vi "g_Joystick2.vi"(7 "Action":enum16{"initialize", "read", "write"}(ring), 9 "Buttons":bool[](array[boolean]), 10 "Axes":dbl[](array[numeric]), 11 "DebounceLength":i32=1) -> (1 "Buttons out":T2, 2 "Axes out":T1 {"Switch" format="%#_4g"; "Axis 2" format="%#_4g"; "Axis 1" format="%#_4g"; "Axis 0" format="%#_4g"}, 4 "Array":cluster{"DbArray":bool[]}[](array[cluster]))   [LabVIEW 2017]
uses:
  Ctrl Refs/JoyStick2.ctl
  Ctrl Refs/JoyStick2(Analog).ctl
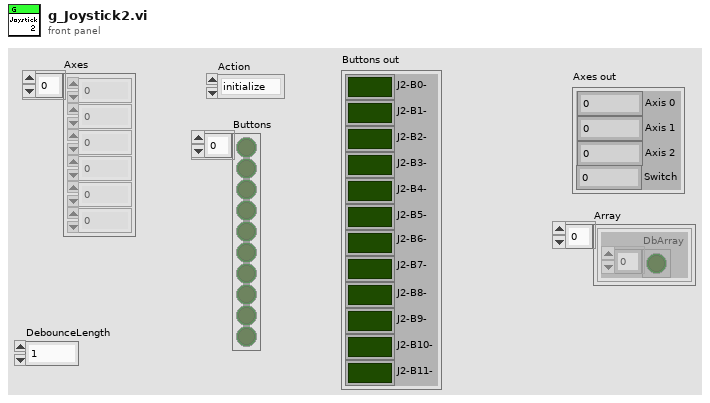
[diagram p1: front panel]
types:
  T1 = typedef "JoyStick2(Analog).ctl" = cluster{"Axis 0":dbl, "Axis 1":dbl, "Axis 2":dbl, "Switch":dbl}
  T2 = typedef "JoyStick2.ctl" = cluster{"J2-B0-":bool, "J2-B1-":bool, "J2-B2-":bool, "J2-B3-":bool, "J2-B4-":bool, "J2-B5-":bool, "J2-B6-":bool, "J2-B7-":bool, "J2-B8-":bool, "J2-B9-":bool, "J2-B10-\n":bool, "J2-B11-":bool}
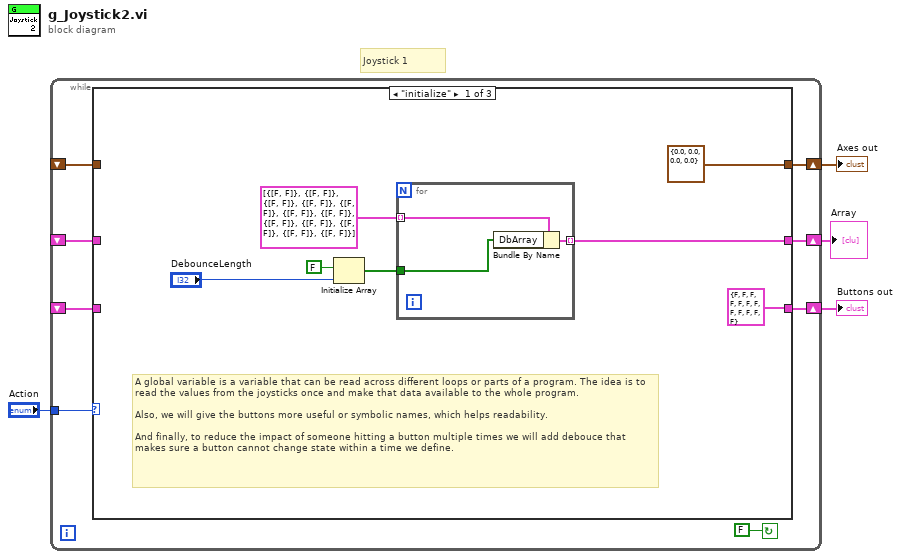
[diagram p0: block diagram]
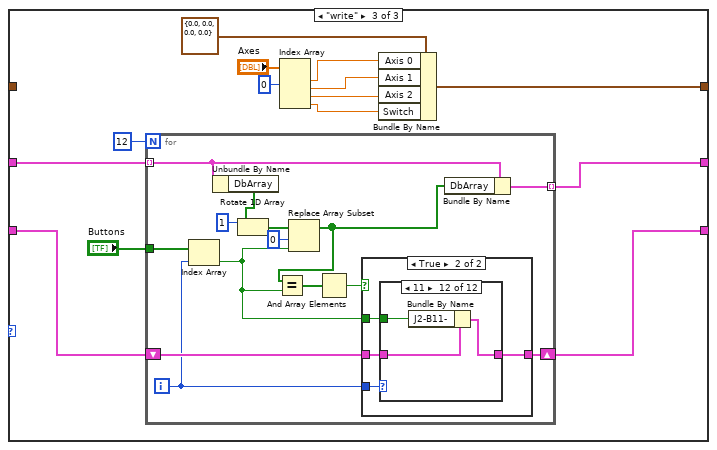
[diagram p3: hidden frame]
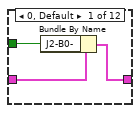
[diagram p5: hidden frame]
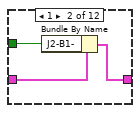
[diagram p6: hidden frame]
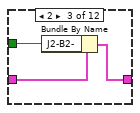
[diagram p7: hidden frame]
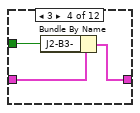
[diagram p8: hidden frame]
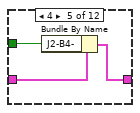
[diagram p9: hidden frame]
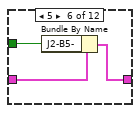
[diagram p10: hidden frame]
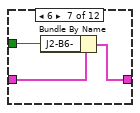
[diagram p11: hidden frame]
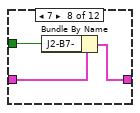
[diagram p12: hidden frame]
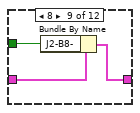
[diagram p13: hidden frame]
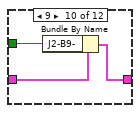
[diagram p14: hidden frame]
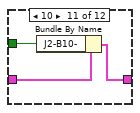
[diagram p15: hidden frame]
diagram:
  # "Joystick 1"
  n1 = while {
    tunnel: "Action" -> [w11]
    shift-right: [w10] -> w2
    shift-left: _ -> [w9]
    shift-right: [w8] -> w3
    shift-left: _ -> [w7]
    shift-right: [w6] -> w1
    shift-left: _ -> [w5]
    stop <- FALSE continue-if-true
    n2 = case shown="\"initialize\"" w11 {
      tunnel: [T1 {"Axis 0"=0.0, "Axis 1"=0.0, "Axis 2"=0.0, "Switch"=0.0} ("Axes out") w25 w35] -> w10
      tunnel: w9 -> [_ w25 _]
      tunnel: [w15 w24 w31] -> w8
      tunnel: w7 -> [_ w24 w32]
      tunnel: [T2 {"J2-B0-"=FALSE, "J2-B1-"=FALSE, "J2-B2-"=FALSE, "J2-B3-"=FALSE, "J2-B4-"=FALSE, "J2-B5-"=FALSE, "J2-B6-"=FALSE, "J2-B7-"=FALSE, "J2-B8-"=FALSE, "J2-B9-"=FALSE, "J2-B10-\n"=FALSE, "J2-B11-"=FALSE} ("Buttons out") w23 w29] -> w6
      tunnel: w5 -> [_ w23 w30]
      frame "initialize" {
        # "A global variable is a variable that can be read across different loops or parts of a program. The idea is to read the values from the joysticks once and make that data available to the whole program.\n \nAlso, we will give the buttons more useful or symbolic names, which helps readability. \n\nAnd finally, to reduce the impact of someone hitting a button multiple times we will add debouce that makes sure a button cannot change state within a time we define."
        n3 = Initialize Array(FALSE, "DebounceLength") -> (w16:bool[])
        n4 = for {
          tunnel: cluster{"DbArray":bool[]}[] [{"DbArray"=[FALSE, FALSE]}, {"DbArray"=[FALSE, FALSE]}, {"DbArray"=[FALSE, FALSE]}, {"DbArray"=[FALSE, FALSE]}, {"DbArray"=[FALSE, FALSE]}, {"DbArray"=[FALSE, FALSE]}, {"DbArray"=[FALSE, FALSE]}, {"DbArray"=[FALSE, FALSE]}, {"DbArray"=[FALSE, FALSE]}, {"DbArray"=[FALSE, FALSE]}, {"DbArray"=[FALSE, FALSE]}, {"DbArray"=[FALSE, FALSE]}] -> [w22] mode=indexing
          tunnel: w16 -> [w21]
          tunnel: [w20] -> w15 mode=indexing
          n5 = Bundle By Name(cluster=w22, "DbArray"=w21) -> (w20:cluster{"DbArray":bool[]})
        }
      }
      frame "read", Default {
      }
      frame "write" {
        n6 = for {
          N: 12 -> [_]
          tunnel: "Buttons" -> [w42]
          tunnel: w32 -> [w53] mode=indexing
          tunnel: [w48] -> w31 mode=indexing
          shift-right: [w45] -> w29
          shift-left: w30 -> [w46]
          i -> [w41]
          n7 = Index Array(array=w42, index=w41) -> (element=w40:bool)
          n8 = Unbundle By Name(w53) -> ("DbArray"=w49:bool[])
          n9 = Rotate 1D Array(1:w49, 2:1 ("n")) -> (0:w51:bool[])
          n10 = Replace Array Subset(array=w51, new element=w40, index=0) -> (w43:bool[])
          n11 = Equal?(x=w43, y=w40) -> (x = y?=w47:bool[])
          n12 = And Array Elements(Boolean array=w47) -> (logical AND=w44:bool)
          n13 = case shown="True" w44 {
            tunnel: w41 -> [_ w58]
            tunnel: w46 -> [w54 w57]
            tunnel: [w54 w56] -> w45
            tunnel: w40 -> [_ w55]
            frame False {
            }
            frame True {
              n14 = case shown="11" w58 {
                tunnel: w57 -> [w61 w64 w67 w70 w73 w76 w79 w82 w85 w88 w91 w94]
                tunnel: [w60 w63 w66 w69 w72 w75 w78 w81 w84 w87 w90 w93] -> w56
                tunnel: w55 -> [w59 w62 w65 w68 w71 w74 w77 w80 w83 w86 w89 w92]
                frame 0, Default {
                  n15 = Bundle By Name(cluster=w61, "J2-B0-"=w59) -> (w60:T2)
                }
                frame 1 {
                  n16 = Bundle By Name(cluster=w64, "J2-B1-"=w62) -> (w63:T2)
                }
                frame 2 {
                  n17 = Bundle By Name(cluster=w67, "J2-B2-"=w65) -> (w66:T2)
                }
                frame 3 {
                  n18 = Bundle By Name(cluster=w70, "J2-B3-"=w68) -> (w69:T2)
                }
                frame 4 {
                  n19 = Bundle By Name(cluster=w73, "J2-B4-"=w71) -> (w72:T2)
                }
                frame 5 {
                  n20 = Bundle By Name(cluster=w76, "J2-B5-"=w74) -> (w75:T2)
                }
                frame 6 {
                  n21 = Bundle By Name(cluster=w79, "J2-B6-"=w77) -> (w78:T2)
                }
                frame 7 {
                  n22 = Bundle By Name(cluster=w82, "J2-B7-"=w80) -> (w81:T2)
                }
                frame 8 {
                  n23 = Bundle By Name(cluster=w85, "J2-B8-"=w83) -> (w84:T2)
                }
                frame 9 {
                  n24 = Bundle By Name(cluster=w88, "J2-B9-"=w86) -> (w87:T2)
                }
                frame 10 {
                  n25 = Bundle By Name(cluster=w91, "J2-B10-"=w89) -> (w90:T2)
                }
                frame 11 {
                  n26 = Bundle By Name(cluster=w94, "J2-B11-"=w92) -> (w93:T2)
                }
              }
            }
          }
          n27 = Bundle By Name(cluster=w53, "DbArray"=w43) -> (w48:cluster{"DbArray":bool[]})
        }
        n28 = Index Array(array="Axes", index #1=0 ("index")) -> (element #1=w38:dbl, element #2=w37:dbl, element #3=w36:dbl, element #4=w26:dbl)  [unwired: 3 in]
        n29 = Bundle By Name(cluster=T1 {"Axis 0"=0.0, "Axis 1"=0.0, "Axis 2"=0.0, "Switch"=0.0} ("Axes out"), "Axis 0"=w38, "Axis 1"=w37, "Axis 2"=w36, "Switch"=w26) -> (w35:T1)
      }
    }
  }
  "Buttons out" <- w1
  "Axes out" <- w2
  "Array" <- w3
